vi "macro_Rotation2d_AngleRad.vi"   [LabVIEW 2019, in "Trajectory_Library.lvlib"]
uses:
  Rotation2d_GetAngleCosSin.vi
  Trajectory_Library.lvlib
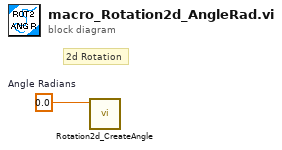
[diagram p0: block diagram]
diagram:
  w1 = 0.0  # Angle Radians
  # "2d Rotation"
  n1 = call "Rotation2d_CreateAngle.vi"("Angle"=w1) -> ()  [unwired: 10 in, 1 out]
